vi "WristDashWriteNetworkSlow.vi"(0 "UseLQR":bool, 4 "FilterDerivative":bool, 6 "Tune_Kg":dbl, 7 "Tune_ErrThres":dbl, 8 "Tune_Kd":dbl, 9 "Tune_OutMax":dbl, 10 "Tune_OutDb":dbl, 11 "Tune_ErrDb":dbl) -> ()   [LabVIEW 2023]
uses:
  <vilib>/Rock Robotics/Network Tables/NT Write Number.vi
  <vilib>/Rock Robotics/Network Tables/NT Write Boolean.vi
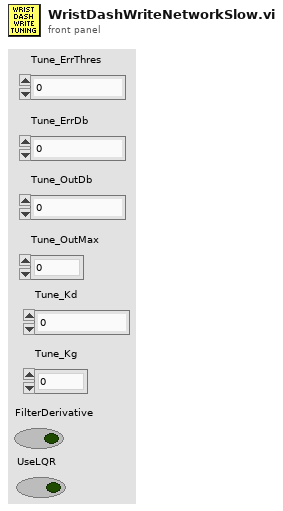
[diagram p1: front panel]
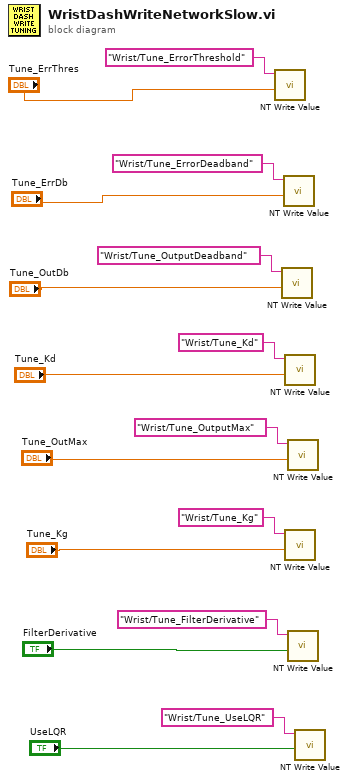
[diagram p0: block diagram]
diagram:
  n1 = call-poly <vilib>:"NT Write Value.vi"("value"="Tune_ErrThres", "name"="Wrist/Tune_ErrorThreshold") -> ()  [unwired: 9 in, 1 out]
  n2 = call-poly <vilib>:"NT Write Value.vi"("value"="Tune_OutDb", "name"="Wrist/Tune_OutputDeadband") -> ()  [unwired: 9 in, 1 out]
  n3 = call-poly <vilib>:"NT Write Value.vi"("value"="Tune_ErrDb", "name"="Wrist/Tune_ErrorDeadband") -> ()  [unwired: 9 in, 1 out]
  n4 = call-poly <vilib>:"NT Write Value.vi"("value"="Tune_Kd", "name"="Wrist/Tune_Kd") -> ()  [unwired: 9 in, 1 out]
  n5 = call-poly <vilib>:"NT Write Value.vi"("value"="Tune_Kg", "name"="Wrist/Tune_Kg") -> ()  [unwired: 9 in, 1 out]
  n6 = call-poly <vilib>:"NT Write Value.vi"("value"="Tune_OutMax", "name"="Wrist/Tune_OutputMax") -> ()  [unwired: 9 in, 1 out]
  n7 = call-poly <vilib>:"NT Write Value.vi"("value"="FilterDerivative", "name"="Wrist/Tune_FilterDerivative") -> ()  [unwired: 9 in, 1 out]
  n8 = call-poly <vilib>:"NT Write Value.vi"("value"="UseLQR", "name"="Wrist/Tune_UseLQR") -> ()  [unwired: 9 in, 1 out]
